vi "Insert Value (Nested Boolean).vi"(7 "key":string[](array[string]), 8 "error in (no error)":errorcluster, 10 "JSON Data in":bool, 11 "JSON Value in":refnum<class "JSON Value.lvclass">) -> (0 "error out":errorcluster, 1 "replaced":bool, 3 "JSON Value out":refnum<class "JSON Value.lvclass">)   [LabVIEW 2016, in "JSON Value.lvclass"]
uses:
  JSON Value.lvclass
  New JSON Value/New JSON Boolean.vi
  Insert Value (Single).vi
  Array/Replace Array Subset/Replace Array Subset (Single).vi
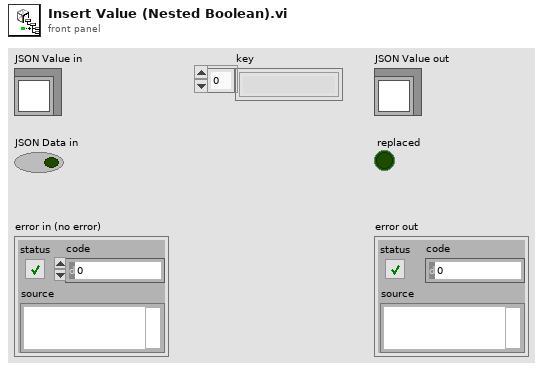
[diagram p1: front panel]
types:
  T1 = typedef "JSON Value.lvclass/JSON Types.ctl" = enum16{"String", "Numeric", "Boolean", "NULL", "Object", "Array"}
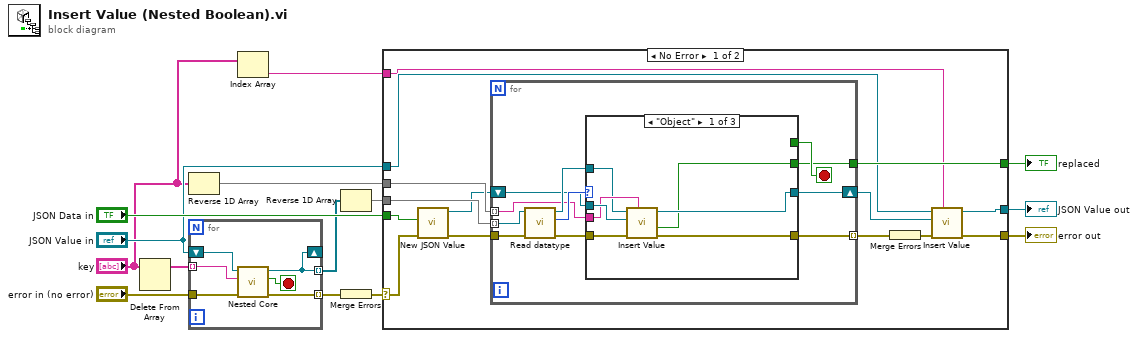
[diagram p0: block diagram]
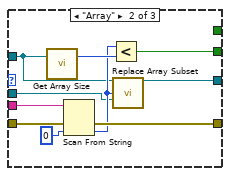
[diagram p2: hidden frame]
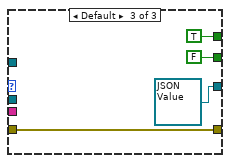
[diagram p3: hidden frame]
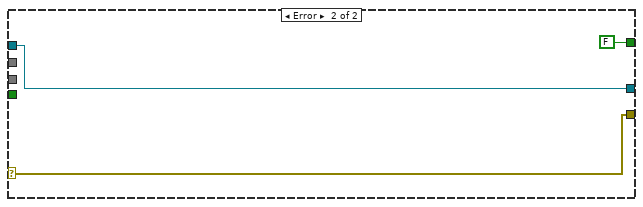
[diagram p4: hidden frame]
diagram:
  n1 = Delete From Array(array="key") -> (array with subset deleted=w10:string[])  [unwired: 2 in, 1 out]
  n2 = Reverse 1D Array(array="key") -> (reversed array=w11:string[])
  n3 = for {
    tunnel: w10 -> [w20] mode=indexing
    shift-right: [w15] -> _
    shift-left: "JSON Value in" -> [w19]
    tunnel: "error in (no error)" -> [w18]
    tunnel: [w17] -> w7 mode=indexing
    tunnel: [w15] -> w8 mode=indexing
    stop <- w16 stop-if-true
    n4 = call "Nested Core.vi"("error in (no error)"=w18, "key"=w20, "JSON Value in"=w19) -> ("error out"=w17:errorcluster, "stop?"=w16:bool, "JSON Value out"=w15:refnum<class "JSON Value.lvclass">)  [unwired: 6 in]
  }
  n5 = Index Array(array="key") -> (element=w1:string)  [unwired: 1 in]
  n6 = Reverse 1D Array(array=w8) -> (reversed array=w12:refnum<class "JSON Value.lvclass">[])
  n7 = Merge Errors(w7) -> (w9:errorcluster)
  n8 = case shown="No Error" w9 {
    selector: w9 -> [w22 w67]
    tunnel: [w34 FALSE ("replaced")] -> w14
    tunnel: "JSON Data in" -> [w24 _]
    tunnel: w12 -> [w33 _]
    tunnel: w11 -> [w32 _]
    tunnel: [w28 w69] -> w4
    tunnel: "JSON Value in" -> [w30 w69]
    tunnel: [w26 w67] -> w3
    tunnel: w1 -> [w25 _]
    frame No Error {
      n9 = call-poly "New JSON Value.vi"("error in (no error)"=w22, "value"=w24) -> ("error out"=w21:errorcluster, "JSON Value out"=w23:refnum<class "JSON Value.lvclass">)  [unwired: 8 in]
      n10 = for {
        tunnel: w32 -> [w37] mode=indexing
        tunnel: w21 -> [w43]
        tunnel: [w42] -> w31 mode=indexing
        tunnel: [w39] -> w34
        tunnel: w33 -> [w38] mode=indexing
        shift-right: [w36] -> w29
        shift-left: w23 -> [w35]
        stop <- w40 stop-if-true
        n11 = call "Read datatype.vi"("error in (no error)"=w43, "JSON Datatype in"=w38) -> ("error out"=w41:errorcluster, "datatype"=w44:T1, "JSON Datatype out"=w45:refnum<class "JSON Value.lvclass">)  [unwired: 7 in]
        n12 = case shown="\"Object\"" w44 {
          tunnel: w37 -> [w48 w57 _]
          tunnel: [w50 w56 refnum<class "JSON Value.lvclass"> refnum ("JSON Object in")] -> w36
          tunnel: w45 -> [w47 w53 _]
          tunnel: [w52 w60 w65] -> w42
          tunnel: w41 -> [w46 w61 w65]
          tunnel: [_ _ TRUE] -> w40
          tunnel: [w49 w58 FALSE] -> w39
          tunnel: w35 -> [w51 w54 _]
          frame "Object" {
            n13 = call-poly "Insert Value.vi"("key"=w48, "error in (no error)"=w46, 10:"JSON Value in"=w51, 11:"JSON Value in"=w47) -> ("error out"=w52:errorcluster, "replaced"=w49:bool, "JSON Value out"=w50:refnum<class "JSON Value.lvclass">)  [unwired: 5 in]
          }
          frame "Array" {
            n14 = call "Get Array Size.vi"("JSON Value in"=w53) -> ("size(s)"=w59:i32)  [unwired: 1 in, 1 out]
            n15 = Scan From String(input string=w57, error in=w61, default 1=0 ("index")) -> (error out=w60:errorcluster, output 1=w55:i32)  [unwired: 2 in, 2 out]
            n16 = Less?(x=w55, y=w59) -> (x < y?=w58:bool)
            n17 = call-poly "Replace Array Subset.vi"("JSON Array"=w53, "index"=w55, "new element/subarray"=w54) -> ("output JSON Array"=w56:refnum<class "JSON Value.lvclass">)  [unwired: 11 in, 1 out]
          }
          frame Default {
          }
        }
      }
      n18 = Merge Errors(w31) -> (w27:errorcluster)
      n19 = call-poly "Insert Value.vi"("key"=w25, "error in (no error)"=w27, 10:"JSON Value in"=w29, 11:"JSON Value in"=w30) -> ("error out"=w26:errorcluster, "JSON Value out"=w28:refnum<class "JSON Value.lvclass">)  [unwired: 5 in, 1 out]
    }
    frame Error {
    }
  }
  "replaced" <- w14
  "error out" <- w3
  "JSON Value out" <- w4
